vi "SPTopLevel.vi"(8 "SetVolt":u32 format="%032b", 9 "heinzingerControl":T1) -> (1 "DACtimeOut":bool)   [LabVIEW 2014]
uses:
  Controls/heinzingerSelect.ctl
  <vilib>/rvi/Emulation/niFpgaGetClockAttributes.vi
  <vilib>/rvi/Emulation/niFpgaSctlEmulationGetInTimedLoop.vi
  <vilib>/rvi/Emulation/niFpgaEmulationReportErrorSimple.vi
  simpleCounterGlobals.vi
  <vilib>/rvi/Emulation/niFpgaProcessEmulError.vi
  <vilib>/rvi/Emulation/niFpgaCriticalErrorInLSC.vi
panel:
  out "simpleCounterWriteOverflow":bool
  in  "stop":bool
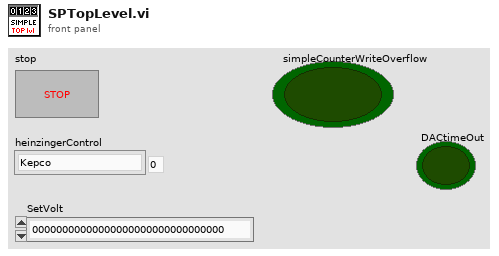
[diagram p1: front panel]
types:
  T1 = typedef "heinzingerSelect.ctl" = enum8{"Kepco", "Heinzinger0", "Heinzinger1", "Heinzinger2"}
  T2 = cluster{"SCLK":refnum<k21>, "CS":refnum<k21>, "MOSI":refnum<k21>, "MISO":refnum<k21>}
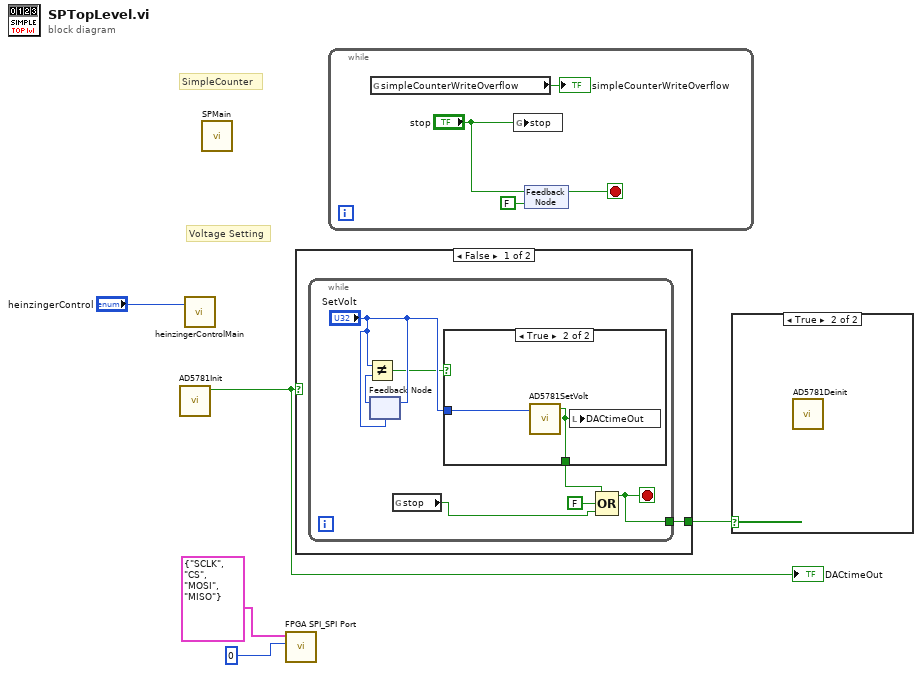
[diagram p0: block diagram]
diagram:
  # "Voltage Setting"
  # "SimpleCounter"
  n1 = call "AD5781Init.vi"() -> ("timeOut"=w3:bool)  [unwired: 11 in]
  "DACtimeOut" <- w3
  n2 = call "heinzingerControlMain.vi"("heinzingerControl"="heinzingerControl") -> ()  [unwired: 2 in]
  n3 = call "SPMain.vi"() -> ()  [unwired: 12 in]
  n4 = call "FPGA SPI_SPI Port.vi"("Port"=i8 0, "FPGA IO"=T2 {"SCLK"="SCLK", "CS"="CS", "MOSI"="MOSI", "MISO"="MISO"}) -> ()  [unwired: 10 in]
  n5 = case shown="False" w3 {
    tunnel: [w6 _] -> w1
    frame False {
      n6 = while {
        tunnel: [w8] -> w6
        stop <- w8 stop-if-true
        n7 = feedback-in #1("SetVolt") -> ()
        n8 = feedback #1("SetVolt") -> (w11:u32)
        n9 = Not Equal?(x="SetVolt", y=w11) -> (x != y?=w9:bool)
        n10 = global read "simpleCounterGlobals.vi" "stop"() -> (w7:bool)
        n11 = case shown="True" w9 {
          tunnel: "SetVolt" -> [_ w15]
          tunnel: [_ w14] -> w12
          frame False {
          }
          frame True {
            n12 = call "AD5781SetVolt.vi"("SetVolt"=w15) -> ("timedOut"=w14:bool)  [unwired: 4 in]
            n13 = local write "DACtimeOut"(w14) -> ()
          }
        }
        n14 = Compound Arithmetic op=OR(w12, FALSE, w7) -> (w8:bool)
      }
    }
    frame True {
    }
  }
  n15 = while {
    stop <- w18 stop-if-true
    n16 = global read "simpleCounterGlobals.vi" "simpleCounterWriteOverflow"() -> (→"simpleCounterWriteOverflow":bool)
    n17 = global write "simpleCounterGlobals.vi" "stop"("stop") -> ()
    n18 = feedback-in #2("stop") -> ()
    n19 = feedback #2(FALSE ("stop")) -> (w18:bool)
  }
  n20 = case shown="True" w1 {
    frame False {
    }
    frame True {
      n21 = call "AD5781Deinit.vi"() -> ()  [unwired: 3 in, 1 out]
    }
  }
